vi "Measure configuration.vi"(0 "Intrument Handle[]":refnum<k15>[](array[refnum]), 1 "Aperture Time":dbl[](array[numeric]), 5 "Channel Name":string[](array[string]), 7 "Measure Period":dbl=0.001 format="%#.3p", 9 "Measurement Configuration":T1={"Quick Power Down"=FALSE, "Pin Name"=[], "Source Mode"=[], "Start Value"=[], "Target Value"=[], "Compliance Limit"=[], "Sense Mode"=[], "Default Ramp Rate"=[], "Ramp Rate"=[], "Start Delay"=[], "Relative To"=[], "Transient Response"=[], "Data Capture"=FALSE, "Power line frequency"=1} {"Power line frequency" items=["50 Hz", "60 Hz"]; "Start Value" format="%#_6p"; "Transient Response" items=["Slow", "Normal", "Fast"]; "Sense Mode" items=["Local Sense", "Remote Sense"]; "Relative To" items=["Power sequence start", "Previous source start", "Previous source end"]; "Target Value" format="%#_6p"; "Source Mode" items=["DC Voltage", "DC Current"]; "Start Delay" format="%#_6p"; "Compliance Limit" format="%#_6p"; "Ramp Rate" format="%#_6p"}, 11 "error in (no error)":errorcluster) -> (4 "Intrument Handle out[]":refnum<k15>[](array[refnum]), 6 "Aperture Time":dbl[](array[numeric]), 15 "error out":errorcluster)   [LabVIEW 2024, in "devicePowerSequencerCoreLogic.lvlib"]
doc: "Measure configurations are done in this VI"
uses:
  devicePowerSequencerCoreLogic.lvlib
  Measurement Configuration.ctl
  controls/Source Mode.ctl
  controls/Sense Mode.ctl
  controls/Relative To.ctl
  controls/Transient Response.ctl
  controls/Power line frequency.ctl
  Device Power Sequencer.lvlib
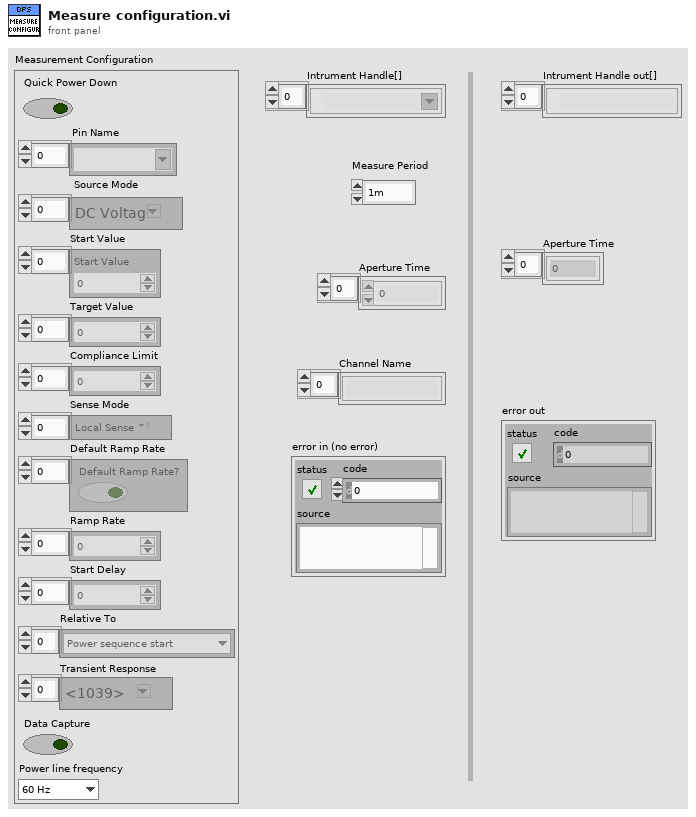
[diagram p1: front panel]
types:
  T1 = typedef "Device Power Sequencer.lvlib/Measurement Configuration.ctl" = cluster{"Quick Power Down":bool, "Pin Name":string[], "Source Mode":T2[], "Start Value":dbl[], "Target Value":dbl[], "Compliance Limit":dbl[], "Sense Mode":T3[], "Default Ramp Rate":bool[], "Ramp Rate":dbl[], "Start Delay":dbl[], "Relative To":T4[], "Transient Response":T5[], "Data Capture":bool, "Power line frequency":T6}
  T2 = typedef "Device Power Sequencer.lvlib/Source Mode.ctl" = i32
  T3 = typedef "Device Power Sequencer.lvlib/Sense Mode.ctl" = i32
  T4 = typedef "Device Power Sequencer.lvlib/Relative To.ctl" = u32
  T5 = typedef "Device Power Sequencer.lvlib/Transient Response.ctl" = i32
  T6 = typedef "Device Power Sequencer.lvlib/Power line frequency.ctl" = u32
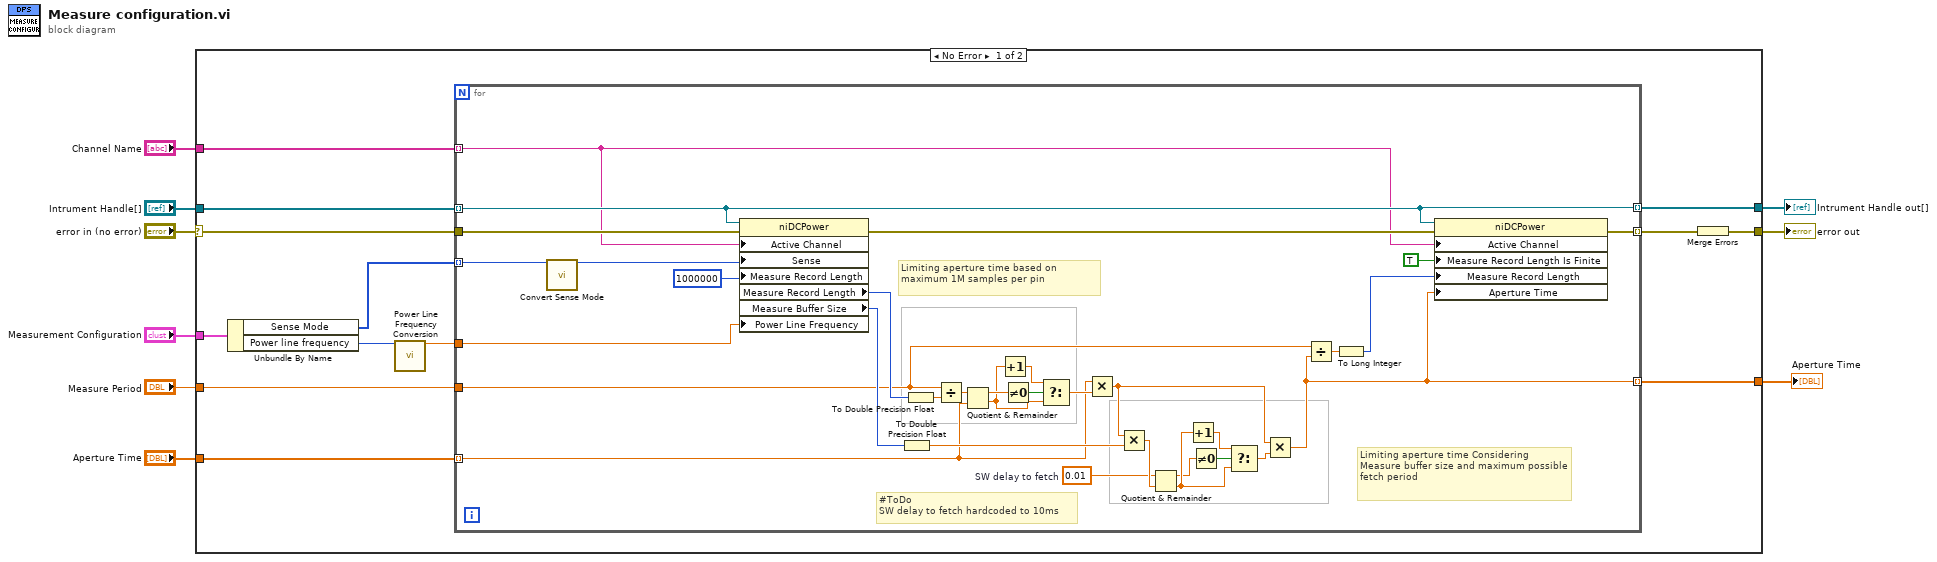
[diagram p0: block diagram]
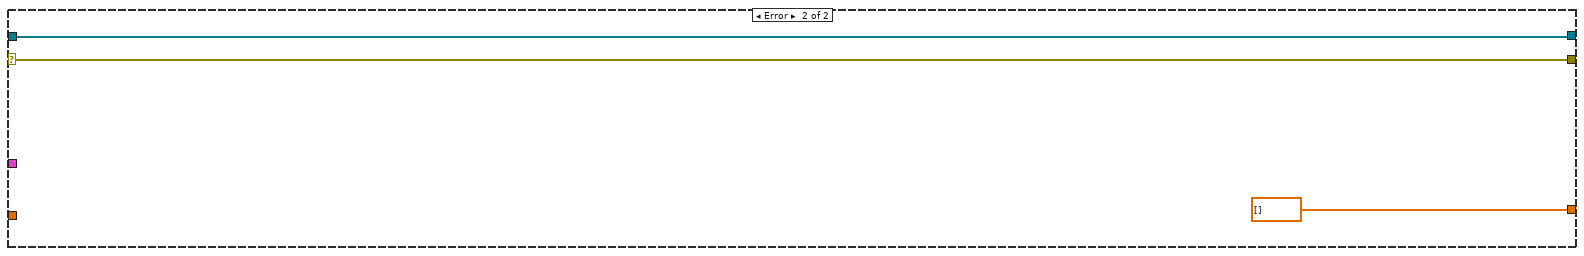
[diagram p2: hidden frame]
diagram:
  n1 = case shown="No Error" "error in (no error)" {
    selector: "error in (no error)" -> [w21 w58]
    tunnel: "Intrument Handle[]" -> [w22 w57]
    tunnel: [w20 w58] -> w7
    tunnel: "Channel Name" -> [w19 _]
    tunnel: "Measure Period" -> [w17 _]
    tunnel: [w16 w57] -> w4
    tunnel: [w15 dbl[] []] -> w3
    tunnel: "Measurement Configuration" -> [w14 _]
    tunnel: "Aperture Time" -> [w12 _]
    frame No Error {
      n2 = Unbundle By Name(w14) -> ("Sense Mode"=w13:T3[], "Power line frequency"=w11:T6)
      n3 = call "Power Line Frequency Conversion.vi"("Power line frequency"=w11) -> ("Power Line Freq"=w10:dbl)  [unwired: 14 in]
      n4 = for {
        tunnel: w22 -> [w46] mode=indexing
        tunnel: w21 -> [w55]
        tunnel: w19 -> [w43] mode=indexing
        tunnel: [w46] -> w16 mode=indexing
        tunnel: [w44] -> w18 mode=indexing
        tunnel: w17 -> [w23]
        tunnel: [w29] -> w15 mode=indexing
        tunnel: w13 -> [w25] mode=indexing
        tunnel: w12 -> [w28] mode=indexing
        tunnel: w10 -> [w26]
        w31 = 0.01  # SW delay to fetch
        # "Limiting aperture time Considering Measure buffer size and maximum possible fetch period"
        # "Limiting aperture time based on maximum 1M samples per pin"
        # "#ToDo\nSW delay to fetch hardcoded to 10ms"
        n5 = call "Convert Sense Mode.vi"("Sense"=w25) -> ("Measurement:Sense"=w24:i32)  [unwired: 14 in]
        n6 = property class="niDCPower"(reference=w46, error in=w55, "Active Channel"=w43, "Sense"=w24, "Measure Record Length"=1000000 ("Measurement:Measure Record Length"), "Power Line Frequency"=w26) -> (error out=w45:errorcluster, "Measure Record Length"=w41:i32, "Measure Buffer Size"=w34:i32)  [unwired: 1 out]
        n7 = To Double Precision Float(number=w34) -> (double precision float=w33:dbl)
        n8 = To Double Precision Float(number=w41) -> (double precision float=w42:dbl)
        n9 = Divide(x=w23, y=w42) -> (x/y=w54:dbl)
        n10 = Quotient & Remainder(x=w54, y=w28) -> (x-y*floor(x/y)=w53:dbl, floor(x/y)=w51:dbl)
        n11 = Increment(x=w51) -> (x+1=w50:dbl)
        n12 = Not Equal To 0?(x=w53) -> (x != 0?=w52:bool)
        n13 = Select(t=w50, s=w52, f=w51) -> (s? t:f=w49:dbl)
        n14 = Multiply(x=w28, y=w49) -> (x*y=w30:dbl)
        n15 = Multiply(x=w30, y=w33) -> (x*y=w32:dbl)
        n16 = Quotient & Remainder(x=w31, y=w32) -> (x-y*floor(x/y)=w35:dbl, floor(x/y)=w37:dbl)
        n17 = Increment(x=w37) -> (x+1=w38:dbl)
        n18 = Not Equal To 0?(x=w35) -> (x != 0?=w36:bool)
        n19 = Select(t=w38, s=w36, f=w37) -> (s? t:f=w39:dbl)
        n20 = Multiply(x=w30, y=w39) -> (x*y=w29:dbl)
        n21 = Divide(x=w23, y=w29) -> (x/y=w48:dbl)
        n22 = To Long Integer(number=w48) -> (32bit integer=w27:i32)
        n23 = property class="niDCPower"(reference=w46, error in=w45, "Active Channel"=w43, "Measure Record Length Is Finite"=TRUE ("Measurement:Measure Record Length Is Finite"), "Measure Record Length"=w27, "Aperture Time"=w29) -> (error out=w44:errorcluster)  [unwired: 1 out]
      }
      n24 = Merge Errors(w18) -> (w20:errorcluster)
    }
    frame Error {
    }
  }
  "error out" <- w7
  "Intrument Handle out[]" <- w4
  "Aperture Time" <- w3
